vi "DialogCreateMethod.vi"(0 "ClassWriter in":refnum<class "ClassWriter.lvclass">, 1 "ClassItemRefIn":refnum<vi>, 5 "error in (no error)":errorcluster) -> (14 "ClassWriter out":refnum<class "ClassWriter.lvclass">, 15 "ClassItemRefOut":refnum<vi>, 16 "CreateMethodData":T1={"MethodName"="", "RelativeMethodPath"=path "", "MethodDescription"="", "Scope/Visibility"=enum."Use Parent Folder Scope", "MethodTemplateName"="", "IconOut"=[], "RelativeProjectClassPath"="", "OpenViAfterCreation"=FALSE, "DynamicDispatchVi"=FALSE, "ExtraCreateParameters"=variant, "MustOverride"=FALSE, "MustCallParent"=FALSE, "IconDetails"={"IconSize"=enum."1 c-term high", "ImageRows(32)"=32, "ConnectorPaneHeight"=[]}, "AF-Option"=variant, "TemplatePath"=path ""} {"IconOut" format="%x"}, 17 "Cancelled":bool, 19 "error out":errorcluster)   [LabVIEW 2014, in "ClassWriter.lvclass"]
uses:
  <resource>/Framework/Providers/Open_GDS/ClassProviders/Provider_BaseClassInterface/ClassWriter_class/ClassWriter.lvclass
  <resource>/Framework/Providers/Open_GDS/ClassProviders/Provider_BaseClassInterface/CreateMethodData.ctl
  <resource>/Framework/Providers/Open_GDS/ClassProviders/Provider_EndevoGOOP300/GOOP300_SubVIs/GOOP300_MethodScopeType.ctl
  <resource>/Framework/Providers/Open_GDS/ClassProviders/Provider_LvNativeClass/ClassWriterNative_class/IconDetails.ctl
  <resource>/Framework/Providers/Open_GDS/ClassProviders/Provider_LvNativeClass/ClassWriterNative_class/IconSize.ctl
  <resource>/Framework/Providers/Open_GDS/ClassProviders/Provider_LvNativeClass/ClassWriterNative_class/ClassWriterNative.lvclass
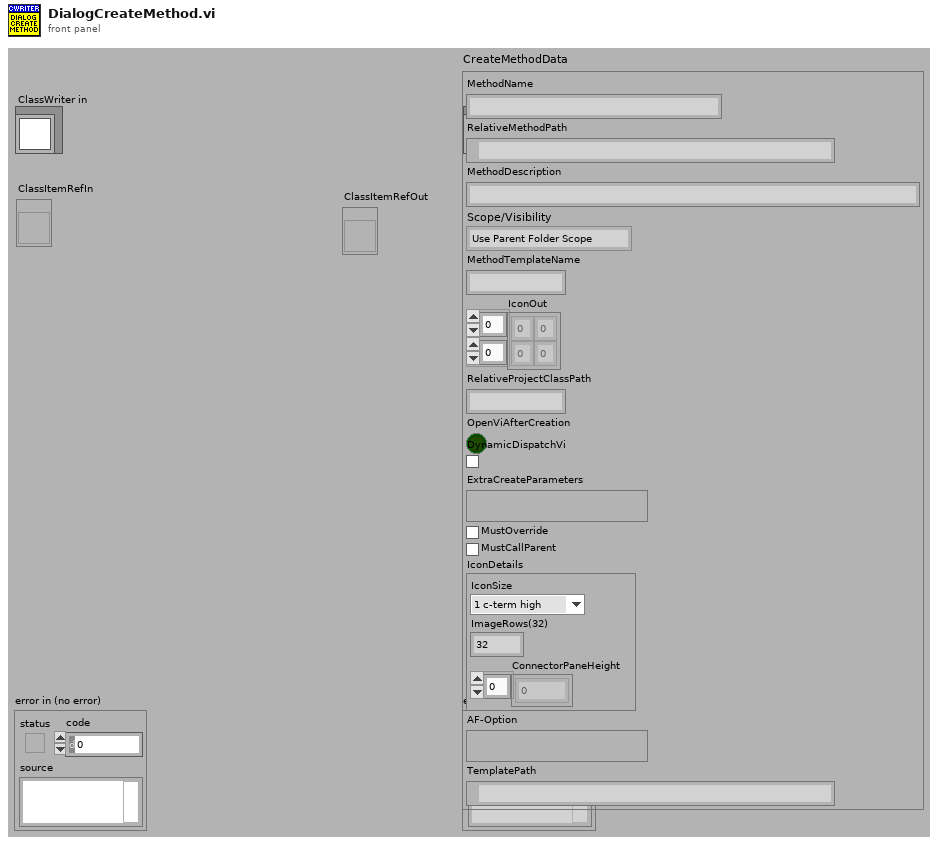
[diagram p1: front panel]
types:
  T1 = typedef "ClassWriter.lvclass/CreateMethodData.ctl" = cluster{"MethodName":string, "RelativeMethodPath":path, "MethodDescription":string, "Scope/Visibility":T2, "MethodTemplateName":string, "IconOut":u8[][], "RelativeProjectClassPath":string, "OpenViAfterCreation":bool, "DynamicDispatchVi":bool, "ExtraCreateParameters":variant, "MustOverride":bool, "MustCallParent":bool, "IconDetails":T3, "AF-Option":variant, "TemplatePath":path}
  T2 = typedef "GOOP300_MethodScopeType.ctl" = enum16{"Use Parent Folder Scope", "Public", "Protected", "Private", "Community"}
  T3 = typedef "ClassWriterNative.lvclass/IconDetails.ctl" = cluster{"IconSize":T4, "ImageRows(32)":i32, "ConnectorPaneHeight":i32[]}
  T4 = typedef "ClassWriterNative.lvclass/IconSize.ctl" = enum16{"Full", "1 c-term high", "2 c-term high", "3 c-term high"}
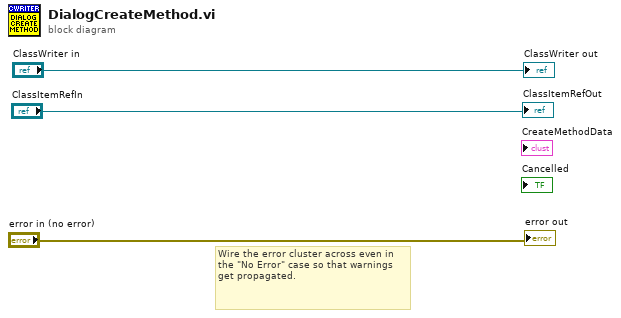
[diagram p0: block diagram]
diagram:
  # "Wire the error cluster across even in the \"No Error\" case so that warnings get propagated."
  "error out" <- "error in (no error)"
  "ClassWriter out" <- "ClassWriter in"
  "ClassItemRefOut" <- "ClassItemRefIn"
